vi "EscribirVoltaje_Ini.vi"(3 "physical channels":tag="Dev1/ao1") -> (0 "error out":errorcluster, 1 "cluster":T1)   [LabVIEW 2017]
uses:
  <vilib>/DAQmx/create/channels.llb/DAQmx Create Channel (AO-Voltage-Basic).vi
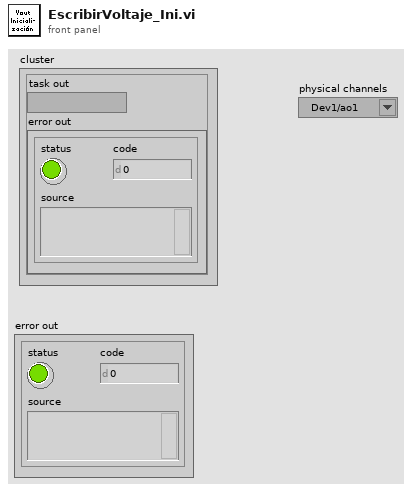
[diagram p1: front panel]
types:
  T1 = cluster{"task out":refnum<k21>, "error out":errorcluster}
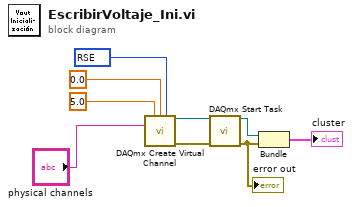
[diagram p0: block diagram]
diagram:
  w7 = 10083 items=["Default"=-1, "RSE"=10083, "Differential"=10106, "Pseudodifferential"=12529] ("output terminal configuration")
  n1 = call-poly <vilib>:"DAQmx Create Virtual Channel.vi"("maximum value"=5.0, "minimum value"=0.0, "output terminal configuration"=w7, "physical channels"="physical channels") -> ("task out"=w3:refnum<k21>, "error out"=w4:errorcluster)  [unwired: 10 in]
  n2 = call <vilib>:"DAQmx Start Task.vi"("task/channels in"=w3, "error in"=w4) -> ("task out"=w8:refnum<k21>, "error out"=w9:errorcluster)  [unwired: 12 in]
  "error out" <- w9
  n3 = Bundle("task out"=w8, "error out"=w9) -> (→"cluster":T1)  [unwired: 1 in]
